vi "DriveScale.vi"(11 "Numeric in":dbl) -> (3 "Numeric out":dbl)   [LabVIEW 2015]
doc: "Here we take the joystick values and divide the the positive values to three intervals.\n0-.33\n.33-.66\n.66-1.0\nand assigng them steady values... Consider making MORE INTERVALS"
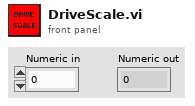
[diagram p1: front panel]
types:
  T1 = typedef "constants.ctl" = cluster{"motorConstants":cluster{"leftDriveMotor":i32, "rightDriveMotor":i32, "climberAngler":i32, "climberWinch":T2, "shooterTopFlyWheel":T2, "shooterBottomFlyWheel":T2, "climberExtender":i32, "shooterIntakeWheel":T2}, "arduinoInputChannel":cluster{"armAngleUp":i32, "intakeWheelSpinIn":i32, "winchUp":i32, "extenderUp":i32, "AimingAuto":i32, "extenderDown":i32}, "driveConstants":cluster{"firstIntervalPercent":dbl, "secondIntervalPercent":dbl, "thirdIntervalPercent":dbl}, "cRioInputChanels":cluster{"photoEye":i32, "limitExtender":i32}, "pneumaticsChannels":cluster{"angleSolenoid":T3, "shooterAnglerPneumatic":T3}, "flyWheelConstants":cluster{"manualTopWheel":dbl, "manualBottomWheel":dbl, "autoFuncConst1":dbl, "autoFuncConst2":dbl, "autoFuncConst3":dbl, "autoFuncConst4":dbl, "Array":dbl[][]}}
  T2 = typedef "FPGA_DIOPWMChannel.ctl" = enum8{"PWM 0", "PWM 1", "PWM 2", "PWM 3", "PWM 4", "PWM 5", "PWM 6", "PWM 7", "PWM 8", "PWM 9", "PWM MXP 0", "PWM MXP 1", "PWM MXP 2", "PWM MXP 3", "PWM MXP 4", "PWM MXP 5", "PWM MXP 6", "PWM MXP 7", "PWM MXP 8", "PWM MXP 9", "Invalid"}
  T3 = typedef "WPI_SolenoidChannel.ctl" = enum8{"Solenoid 0", "Solenoid 1", "Solenoid 2", "Solenoid 3", "Solenoid 4", "Solenoid 5", "Solenoid 6", "Solenoid 7", "Invalid"}
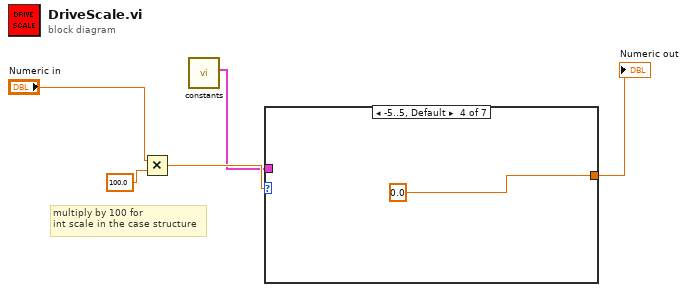
[diagram p0: block diagram]
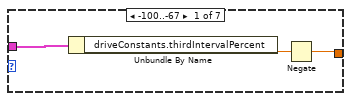
[diagram p2: hidden frame]
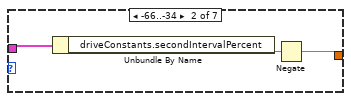
[diagram p3: hidden frame]
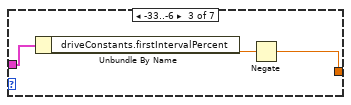
[diagram p4: hidden frame]
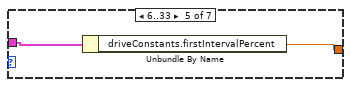
[diagram p5: hidden frame]
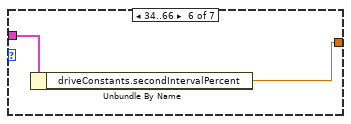
[diagram p6: hidden frame]
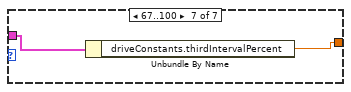
[diagram p7: hidden frame]
diagram:
  # "multiply by 100 for \nint scale in the case structure"
  n1 = Multiply(x="Numeric in", y=100.0) -> (x*y=w2:dbl)
  n2 = call "constants.vi"() -> (2:w1:T1)  [unwired: 11 in]
  n3 = case shown="-5..5, Default" w2 {
    tunnel: [w6 w9 w13 0.0 w17 w19 w20] -> w5
    tunnel: w1 -> [w8 w10 w12 _ w16 w18 w21]
    frame -100..-67 {
      n4 = Unbundle By Name(w8) -> ("driveConstants.thirdIntervalPercent"=w7:dbl)
      n5 = Negate(x=w7) -> (-x=w6:dbl)
    }
    frame -66..-34 {
      n6 = Unbundle By Name(w10) -> ("driveConstants.secondIntervalPercent"=w11:dbl)
      n7 = Negate(x=w11) -> (-x=w9:dbl)
    }
    frame -33..-6 {
      n8 = Unbundle By Name(w12) -> ("driveConstants.firstIntervalPercent"=w14:dbl)
      n9 = Negate(x=w14) -> (-x=w13:dbl)
    }
    frame -5..5, Default {
    }
    frame 6..33 {
      n10 = Unbundle By Name(w16) -> ("driveConstants.firstIntervalPercent"=w17:dbl)
    }
    frame 34..66 {
      n11 = Unbundle By Name(w18) -> ("driveConstants.secondIntervalPercent"=w19:dbl)
    }
    frame 67..100 {
      n12 = Unbundle By Name(w21) -> ("driveConstants.thirdIntervalPercent"=w20:dbl)
    }
  }
  "Numeric out" <- w5
